vi "Arthur_Q1_VF.vi"() -> ()   [LabVIEW 2019]
uses:
  <vilib>/measure/matone.llb/Extract Single Tone Information 1 Chan.vi
  <vilib>/measure/matone.llb/Extract Multiple Tone Information 1 Chan.vi
  <vilib>/measure/NI_MAPro.lvlib
panel:
  out "?":string="SATISFAZ OS CRITÉRIOS"
  out "DHT":dbl
  in  "Path - Q1":path
  out "Sinal completo":waveform(dbl)(graph)
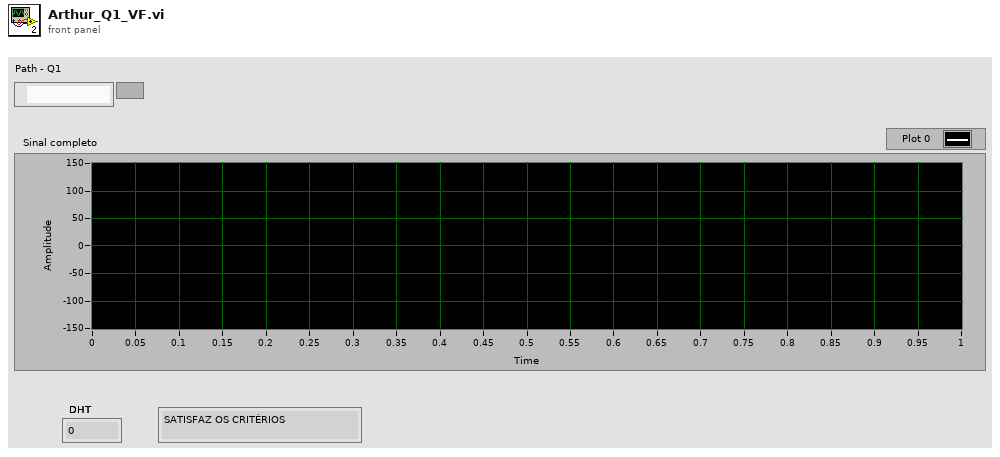
[diagram p1: front panel]
types:
  T1 = cluster{"detected frequency":dbl, "detected amplitude":dbl, "detected phase (deg)":dbl}[]
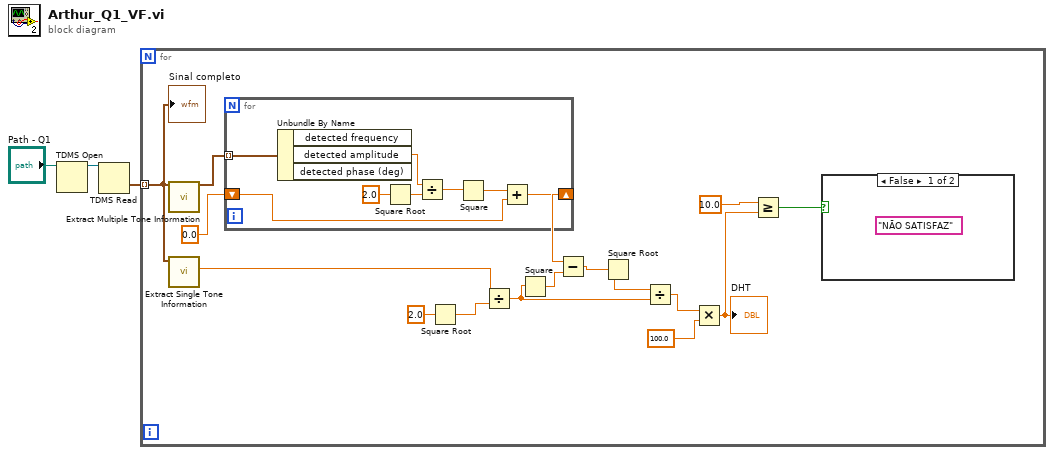
[diagram p0: block diagram]
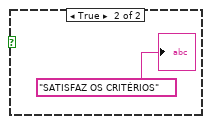
[diagram p2: hidden frame]
diagram:
  n1 = TDMS Open(11:"Path - Q1") -> (3:w3:refnum<k34>)  [unwired: 6 in, 1 out]
  n2 = TDMS Read(0:w3) -> (10:w2:waveform(dbl)[])  [unwired: 7 in, 5 out]
  n3 = for {
    tunnel: w2 -> [w17] mode=indexing
    n4 = call-poly <vilib>:"Extract Multiple Tone Information.vi"("time signal in"=w17) -> ("multiple tone information"=w19:T1)  [unwired: 12 in, 2 out]
    n5 = call-poly <vilib>:"Extract Single Tone Information.vi"("time signal in"=w17) -> ("detected amplitude"=w14:dbl)  [unwired: 5 in, 5 out]
    n6 = for {
      tunnel: w19 -> [w28] mode=indexing
      shift-right: [w21] -> w12
      shift-left: 0.0 -> [w23]
      n7 = Unbundle By Name(w28) -> ("detected amplitude"=w27:dbl)  [unwired: 2 out]
      n8 = Square Root(x=2.0) -> (sqrt(x)=w26:dbl)
      n9 = Divide(x=w27, y=w26) -> (x/y=w25:dbl)
      n10 = Square(x=w25) -> (x^2=w22:dbl)
      n11 = Add(x=w22, y=w23) -> (x+y=w21:dbl)
    }
    n12 = Square Root(x=2.0) -> (sqrt(x)=w15:dbl)
    n13 = Divide(x=w14, y=w15) -> (x/y=w10:dbl)
    n14 = Square(x=w10) -> (x^2=w13:dbl)
    n15 = Subtract(x=w12, y=w13) -> (x-y=w11:dbl)
    n16 = Square Root(x=w11) -> (sqrt(x)=w7:dbl)
    n17 = Divide(x=w7, y=w10) -> (x/y=w9:dbl)
    n18 = Multiply(x=w9, y=100.0) -> (x*y=w6:dbl)
    "DHT" <- w6
    n19 = Greater Or Equal?(x=10.0, y=w6) -> (x >= y?=w4:bool)
    n20 = case shown="False" w4 {
      frame False {
        (unwired) "NÃO SATISFAZ"
      }
      frame True {
        "?" <- "SATISFAZ OS CRITÉRIOS"
      }
    }
    "Sinal completo" <- w17
  }
